vi "path.vi"() -> ()   [LabVIEW 2014]
panel:
  out "添加的路径":path
  out "数组":string[][](array[string])
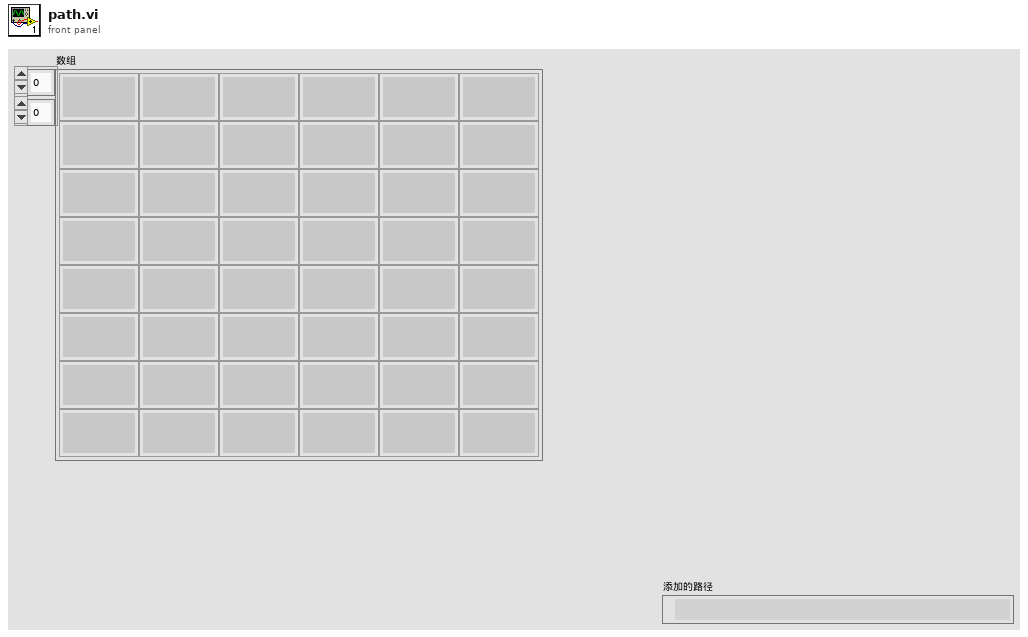
[diagram p1: front panel]
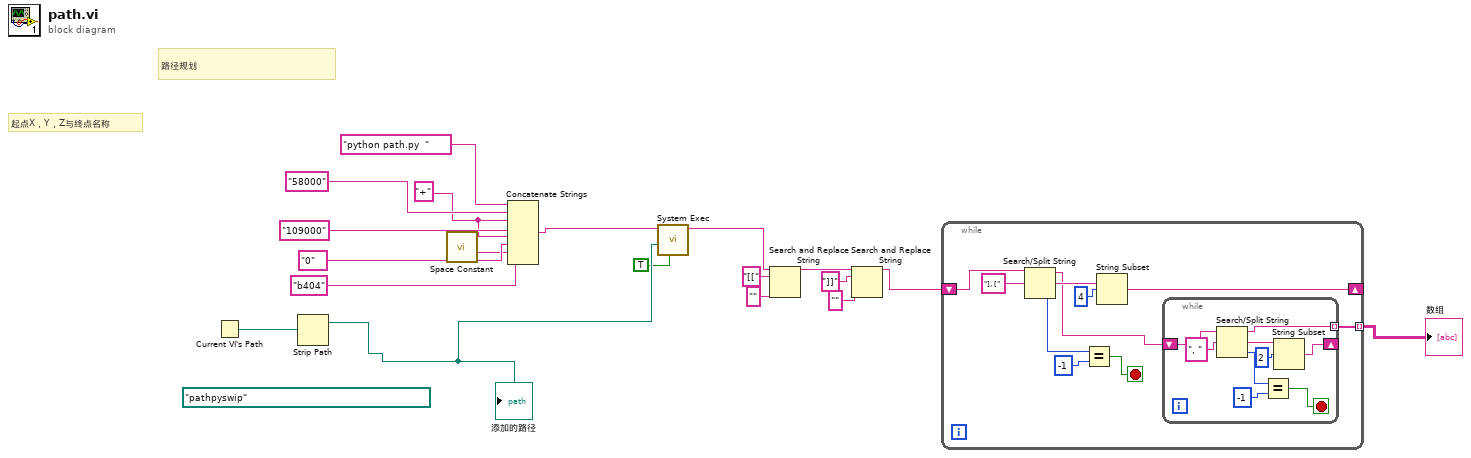
[diagram p0: block diagram]
diagram:
  w2 = "+"
  (unwired) path "pathpyswip"
  # "起点X，Y，Z与终点名称"
  # "路径规划"
  n1 = Current VI's Path() -> (path=w13:path)
  n2 = Strip Path(path=w13) -> (stripped path=w12:path)  [unwired: 1 out]
  "添加的路径" <- w12
  n3 = call <vilib>:"Space Constant.vi"() -> ("String"=w1:string)
  n4 = Concatenate Strings("python path.py  " ("command line"), "58000" ("元素"), w2, "109000" ("元素"), w2, "0" ("元素"), w1, "b404" ("元素")) -> (w14:string)
  n5 = call <vilib>:"System Exec.vi"("run minimized? (F)"=TRUE, "working directory"=w12, "command line"=w14) -> ("standard output"=w3:string)  [unwired: 5 in, 3 out]
  n6 = Search and Replace String(input string=w3, search string="[[" ("搜索字符串"), replace string="" ("替换字符串(\"\")")) -> (result string=w9:string)  [unwired: 5 in, 3 out]
  n7 = Search and Replace String(input string=w9, search string="]]" ("搜索字符串"), replace string="" ("替换字符串(\"\")")) -> (result string=w7:string)  [unwired: 5 in, 3 out]
  n8 = while {
    shift-right: [w25] -> _
    shift-left: w7 -> [w29]
    tunnel: [w21] -> w6 mode=indexing
    stop <- w20 stop-if-true
    n9 = Search/Split String(string=w29, search string/char (-)="], [" ("搜索字符串")) -> (substring before match=w22:string, match + rest of string=w27:string, offset of match=w24:i32)  [unwired: 1 in]
    n10 = Equal?(x=w24, y=-1) -> (x = y?=w20:bool)
    n11 = String Subset(string=w27, offset (0)=4 ("偏移量(0)")) -> (substring=w25:string)  [unwired: 1 in]
    n12 = while {
      shift-right: [w35] -> _
      shift-left: w22 -> [w38]
      tunnel: [w33] -> w21 mode=indexing
      stop <- w30 stop-if-true
      n13 = Search/Split String(string=w38, search string/char (-)=", " ("搜索字符串/字符(-)")) -> (substring before match=w33:string, match + rest of string=w34:string, offset of match=w31:i32)  [unwired: 1 in]
      n14 = Equal?(x=w31, y=-1) -> (x = y?=w30:bool)
      n15 = String Subset(string=w34, offset (0)=2 ("偏移量(0)")) -> (substring=w35:string)  [unwired: 1 in]
    }
  }
  "数组" <- w6
